vi "GetVariablesValues .vi"(8 "error in (no error)":errorcluster, 11 "Sequence Context In":refnum<k7>) -> (0 "error out (no error)":errorcluster, 1 "isInitialLogIn":bool, 2 "LeftCoordinates":i16, 3 "TopCoordinates":i16)   [LabVIEW 2021]
uses:
  <vilib>/addons/TestStand/_TSUtility.llb/TestStand - Get Property Value (Number {Signed 16-bit Integer}).vi
  <vilib>/addons/TestStand/_TSUtility.llb/TestStand - Get Property Value (Boolean).vi
panel:
  out "Sequence Context Out":refnum<k7>
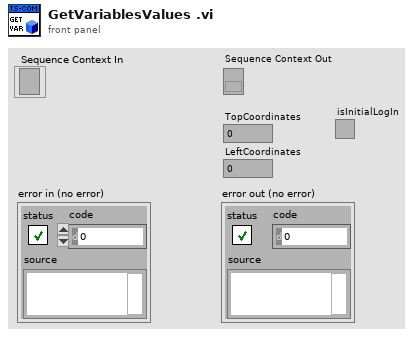
[diagram p1: front panel]
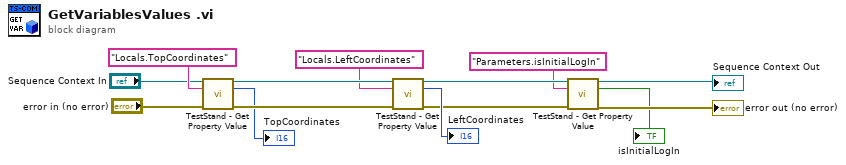
[diagram p0: block diagram]
diagram:
  n1 = call-poly <vilib>:"TestStand - Get Property Value.vi"("Sequence Context In"="Sequence Context In", "Lookup String"="Locals.TopCoordinates", "error in (no error)"="error in (no error)") -> ("Sequence Context Out"=w12:refnum<k7>, "Value"=→"TopCoordinates":i16, "error out"=w11:errorcluster)  [unwired: 10 in]
  n2 = call-poly <vilib>:"TestStand - Get Property Value.vi"("Sequence Context In"=w12, "Lookup String"="Locals.LeftCoordinates", "error in (no error)"=w11) -> ("Sequence Context Out"=w6:refnum<k7>, "Value"=→"LeftCoordinates":i16, "error out"=w7:errorcluster)  [unwired: 10 in]
  n3 = call-poly <vilib>:"TestStand - Get Property Value.vi"("Sequence Context In"=w6, "Lookup String"="Parameters.isInitialLogIn", "error in (no error)"=w7) -> ("Sequence Context Out"=→"Sequence Context Out":refnum<k7>, "Value"=→"isInitialLogIn":bool, "error out"=→"error out (no error)":errorcluster)  [unwired: 10 in]
